vi "Local UV Led Example.vi"() -> ()   [LabVIEW 8.6]
uses:
  TypeDef/UVLed_mode.ctl
  TypeDef/UVLed_channel.ctl
panel:
  in  "expose_sec":dbl
  in  "intrupt":bool
  in  "CHN":T1 items=["All", "CH1", "CH2", "CH3", "CH4"]
  out "Active":bool
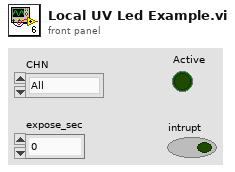
[diagram p1: front panel]
types:
  T1 = typedef "UVLed_channel.ctl" = u16
  T2 = typedef "UVLed_mode.ctl" = u16
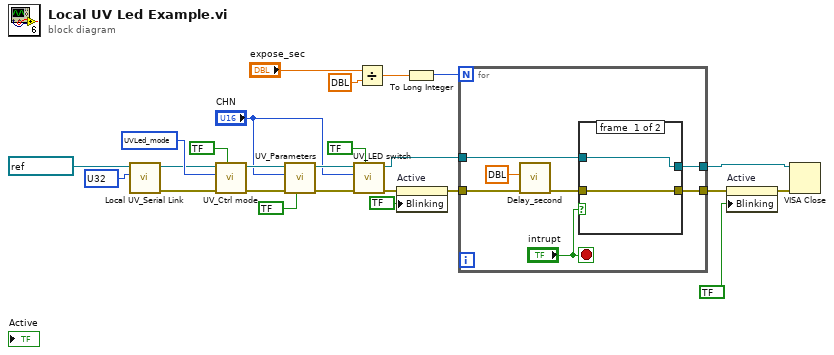
[diagram p0: block diagram]
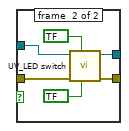
[diagram p2: hidden frame]
diagram:
  w24 = T2 ? items=["MANU", "AUTO", "MANUPRO", "AUTOPRO"] ("Mode")
  n1 = call "Local UV_Serial Link.vi"("baud rate (9600)"=u32 ?, "VISA resource name"=refnum<visa-resource-name> ?) -> ("error out"=w22:errorcluster, "VISA resource out"=w23:refnum<visa-resource-name>)  [unwired: 8 in]
  n2 = call "UV_Ctrl mode.vi"("R/W (F:read)"=bool ?, "error in (no error)"=w22, "Mode"=w24, "VISA resource"=w23) -> ("error out"=w17:errorcluster, "VISA resource out"=w21:refnum<visa-resource-name>)  [unwired: 4 in, 2 out]
  n3 = call "UV_Parameters.vi"("A/M (F:auto)"=bool ?, "error in"=w17, "CHN"="CHN", "VISA resource"=w21) -> ("error out"=w14:errorcluster, "VISA resource out"=w13:refnum<visa-resource-name>)  [unwired: 4 in, 2 out]
  n4 = call "UV_LED switch.vi"("On/Off (F:off)"=bool ?, "error in"=w14, "CHN"="CHN", "VISA resource"=w13) -> ("error out"=w10:errorcluster, "VISA resource out"=w12:refnum<visa-resource-name>)  [unwired: 4 in, 2 out]
  n5 = Divide(x="expose_sec", y=dbl ?) -> (x/y=w3:dbl)
  n6 = property on="Active" class="Bool (strict)"(error in=w10, "Blinking"=bool ?) -> (error out=w6:errorcluster)  [unwired: 1 in, 1 out]
  n7 = To Long Integer(number=w3) -> (32bit integer=w2:i32)
  n8 = for {
    N: w2 -> [_]
    tunnel: w12 -> [w27]
    tunnel: [w30] -> w5
    tunnel: w6 -> [w28]
    tunnel: [w26] -> w11
    stop <- "intrupt" stop-if-true
    n9 = call "Delay_second.vi"("Delay"=dbl ?, "error in (no error)"=w28) -> ("error out"=w31:errorcluster)  [unwired: 8 in]
    n10 = case shown="True" "intrupt" {
      tunnel: w31 -> [w34 w38]
      tunnel: [w34 w37] -> w30
      tunnel: w27 -> [w33 w36]
      tunnel: [w33 w35] -> w26
      frame #0 {
      }
      frame #1 {
        n11 = call "UV_LED switch.vi"("ForceOff"=bool ?, "On/Off (F:off)"=bool ?, "error in"=w38, "VISA resource"=w36) -> ("error out"=w37:errorcluster, "VISA resource out"=w35:refnum<visa-resource-name>)  [unwired: 4 in, 2 out]
      }
    }
  }
  n12 = property on="Active" class="Bool (strict)"(error in=w5, "Blinking"=bool ?) -> (error out=w4:errorcluster)  [unwired: 1 in, 1 out]
  n13 = VISA Close(VISA resource name=w11, error in (no error)=w4) -> ()  [unwired: 1 out]
